vi "MTMount_getNextSample_azimuth.vi"(8 "error in (no error)":errorcluster, 11 "azimuth_Ctl":T1) -> (0 "error out":errorcluster, 2 "function return":i32, 3 "azimuth_Ctl out":T1)   [LabVIEW 2018, in "SALLV_MTMount.lvlib"]
doc: "int MTMount_shm_getNextSample_azimuthLV(MTMount_azimuthLV *azimuth_Ctl );"
uses:
  DataTypes/azimuth.ctl
  SALLV_MTMount.lvlib
  SALLV_MTMount.so
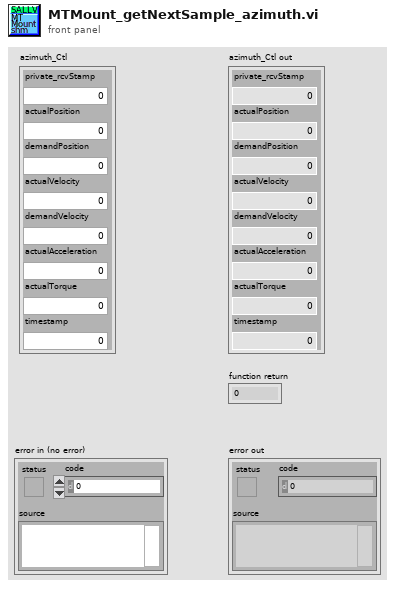
[diagram p1: front panel]
types:
  T1 = typedef "SALLV_MTMount.lvlib/azimuth.ctl" = cluster{"private_rcvStamp":dbl, "actualPosition":dbl, "demandPosition":dbl, "actualVelocity":dbl, "demandVelocity":dbl, "actualAcceleration":dbl, "actualTorque":dbl, "timestamp":dbl}
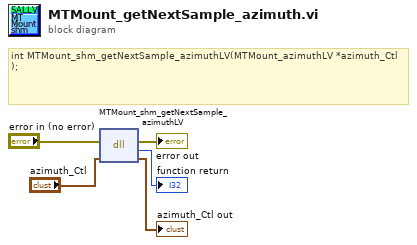
[diagram p0: block diagram]
diagram:
  # "int MTMount_shm_getNextSample_azimuthLV(MTMount_azimuthLV *azimuth_Ctl );"
  n1 = dll-call lib="home/ttsai/Documents/salLabviewApi/SALLV_MTMount/SALLV_MTMount.*" fn="MTMount_shm_getNextSample_azimuthLV"(error in="error in (no error)", "azimuth_Ctl"="azimuth_Ctl") -> (error out=→"error out":errorcluster, →"function return":i32, "azimuth_Ctl"=→"azimuth_Ctl out":T1)  [unwired: 2 in, 1 out]
